vi "Calibrate total steps.vi"(8 "error in (no error)":errorcluster, 9 "Step Amplitude":i32=35, 10 "Axis Number":i32, 11 "Agilis in":T1) -> (0 "error out":errorcluster, 2 "Total Steps":i32, 3 "Agilis out":T1)   [LabVIEW 2016, in "Drivers.lvlib" / "Agilis.lvlib"]
uses:
  Agilis.lvlib
  AgilisCmdLib Refnum.ctl
  D:/Trace Grabber/Drivers/Agilis/AgilisCmdLib.dll
  AgilisCmdLib.dll
  Direction.ctl
  Jog Mode.ctl
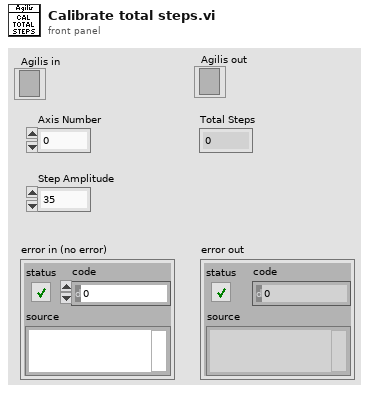
[diagram p1: front panel]
types:
  T1 = typedef "Drivers.lvlib/Agilis.lvlib/AgilisCmdLib Refnum.ctl" = refnum<k24>
  T2 = typedef "Drivers.lvlib/Agilis.lvlib/Jog Mode.ctl" = i32
  T3 = typedef "Drivers.lvlib/Agilis.lvlib/Direction.ctl" = u8
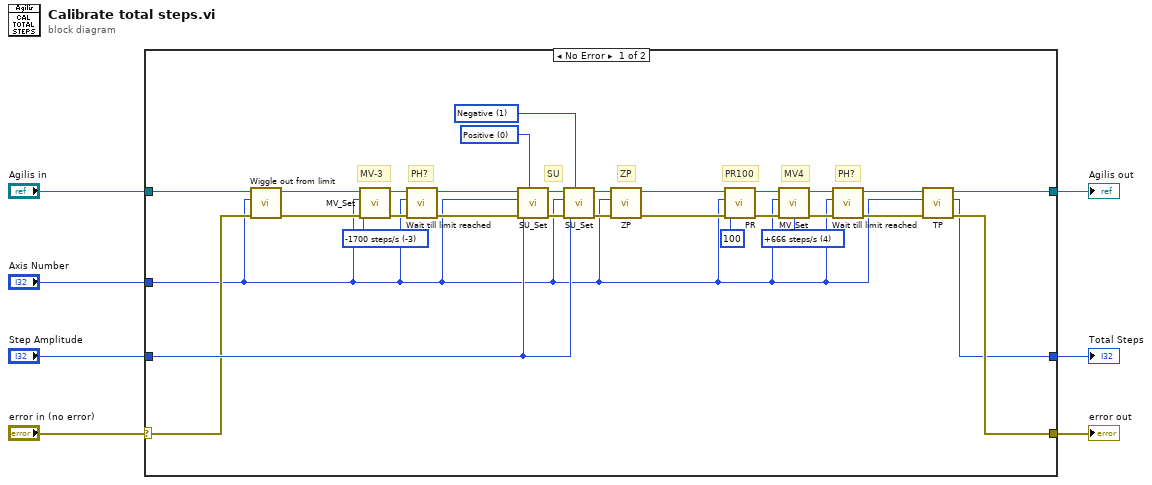
[diagram p0: block diagram]
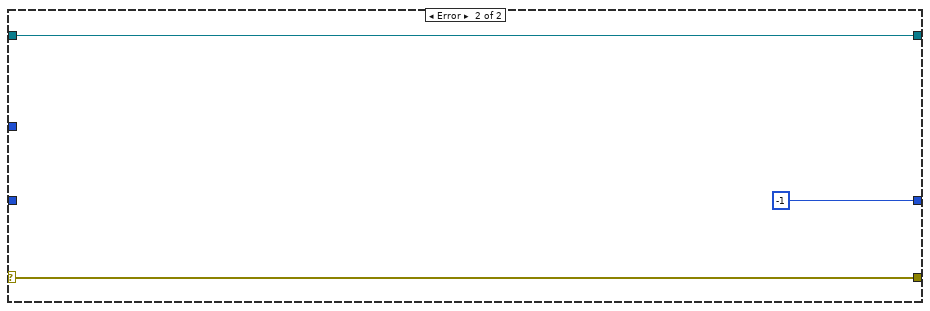
[diagram p2: hidden frame]
diagram:
  n1 = case shown="No Error" "error in (no error)" {
    selector: "error in (no error)" -> [w14 w39]
    tunnel: "Agilis in" -> [w17 w40]
    tunnel: [w22 w40] -> w5
    tunnel: [w20 w39] -> w4
    tunnel: "Axis Number" -> [w9 _]
    tunnel: "Step Amplitude" -> [w19 _]
    tunnel: [w18 -1 ("Accumulated Steps")] -> w1
    frame No Error {
      w26 = T2 4 items=["-666 steps/s"=-4, "-1700 steps/s"=-3, "-100 steps/s"=-2, "-5 steps/s"=-1, "No move"=0, "+5 steps/s"=1, "+100 steps/s"=2, "+1700 steps/s"=3, "+666 steps/s"=4] ("Jog Mode")
      w33 = T2 -3 items=["-666 steps/s"=-4, "-1700 steps/s"=-3, "-100 steps/s"=-2, "-5 steps/s"=-1, "No move"=0, "+5 steps/s"=1, "+100 steps/s"=2, "+1700 steps/s"=3, "+666 steps/s"=4] ("Jog Mode")
      w35 = T3 1 items=["Positive", "Negative"] ("Direction")
      w36 = T3 0 items=["Positive", "Negative"] ("Direction")
      # "PR100"
      # "PH?"
      # "MV4"
      # "ZP"
      # "SU"
      # "PH?"
      # "MV-3"
      n2 = call "Wiggle out from limit.vi"("error in (no error)"=w14, "Axis Number"=w9, "Agilis in"=w17) -> ("error out"=w15:errorcluster, "Agilis out"=w16:T1)  [unwired: 7 in]
      n3 = call "MV_Set.vi"("error in (no error)"=w15, "Jog Mode"=w33, "Axis Number"=w9, "Agilis in"=w16) -> ("error out"=w32:errorcluster, "Agilis out"=w31:T1)  [unwired: 6 in]
      n4 = call "Wait till limit reached.vi"("error in (no error)"=w32, "Axis Number"=w9, ".NET Refnum in"=w31) -> ("error out"=w29:errorcluster, ".NET Refnum out"=w30:T1)  [unwired: 7 in]
      n5 = call "SU_Set.vi"("Direction"=w36, "error in (no error)"=w29, "Step Amplitude"=w19, "Axis Number"=w9, "Agilis in"=w30) -> ("error out"=w34:errorcluster, "Agilis out"=w37:T1)  [unwired: 5 in]
      n6 = call "SU_Set.vi"("Direction"=w35, "error in (no error)"=w34, "Step Amplitude"=w19, "Axis Number"=w9, "Agilis in"=w37) -> ("error out"=w28:errorcluster, "Agilis out"=w27:T1)  [unwired: 5 in]
      n7 = call "ZP.vi"("error in (no error)"=w28, "Axis Number"=w9, "Agilis in"=w27) -> ("error out"=w13:errorcluster, "Agilis out"=w10:T1)  [unwired: 7 in]
      n8 = call "PR.vi"("error in (no error)"=w13, "Target Position"=i64 100, "Axis Number"=w9, "Agilis in"=w10) -> ("error out"=w12:errorcluster, "Agilis out"=w11:T1)  [unwired: 6 in]
      n9 = call "MV_Set.vi"("error in (no error)"=w12, "Jog Mode"=w26, "Axis Number"=w9, "Agilis in"=w11) -> ("error out"=w25:errorcluster, "Agilis out"=w24:T1)  [unwired: 6 in]
      n10 = call "Wait till limit reached.vi"("error in (no error)"=w25, "Axis Number"=w9, ".NET Refnum in"=w24) -> ("error out"=w21:errorcluster, ".NET Refnum out"=w23:T1)  [unwired: 7 in]
      n11 = call "TP.vi"("error in (no error)"=w21, "Axis Number"=w9, "Agilis in"=w23) -> ("error out"=w20:errorcluster, "Accumulated Steps"=w18:i32, "Agilis out"=w22:T1)  [unwired: 6 in]
    }
    frame Error {
    }
  }
  "error out" <- w4
  "Agilis out" <- w5
  "Total Steps" <- w1
